vi "Initialize Sessions.vi"(0 "Session Handle in":T1, 5 "Baud Rate":u32=250000, 7 "Termination":u32(ring)=1 items=["Off", "On"], 11 "error in (no error)":errorcluster) -> (4 "Session Handle Out":T1, 15 "error out":errorcluster)   [LabVIEW 2015, in "PAS.lvclass"]
uses:
  PAS.lvclass
  Typedefs/Session Handle.ctl
  PAS.lvclass/PAS.ctl
  <vilib>/xnet/xnet.llb/XNET Create Session (Frame Output Stream).vi
  <vilib>/xnet/xnet.llb/XNET Create Session (Frame Input Stream).vi
  <resource>/objmgr/xnet.rc
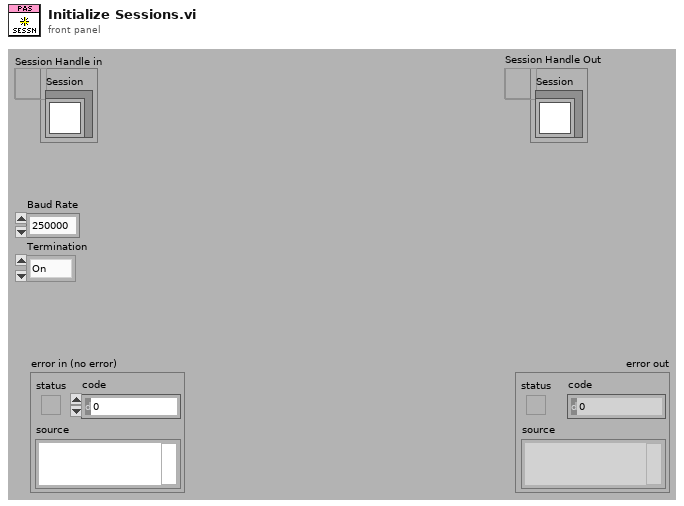
[diagram p1: front panel]
types:
  T1 = typedef "PAS.lvclass/Session Handle.ctl" = refnum<data-value>
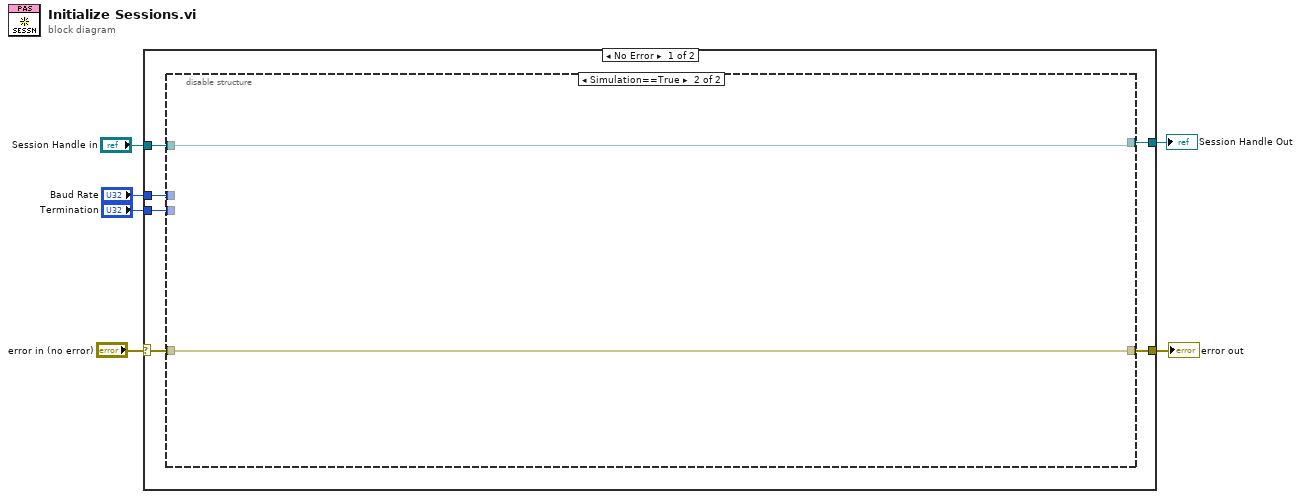
[diagram p0: block diagram]
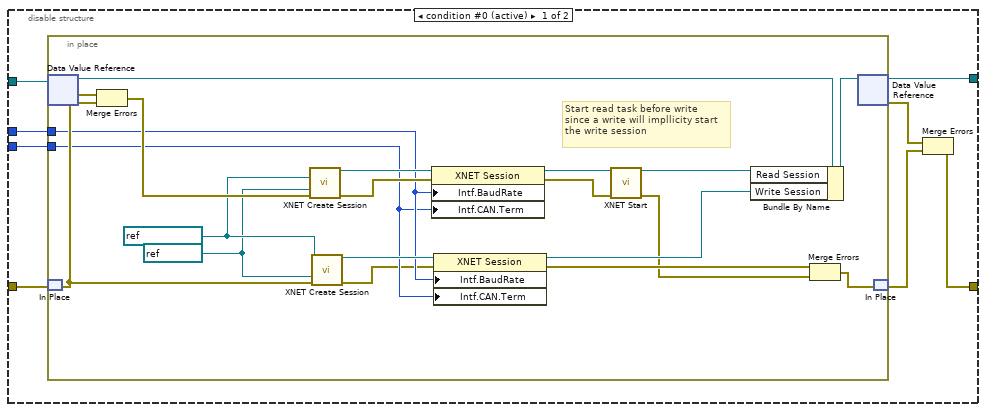
[diagram p2: hidden frame]
diagram:
  n1 = case shown="No Error" "error in (no error)" {
    selector: "error in (no error)" -> [w11 w44]
    tunnel: [w12 w44] -> w6
    tunnel: "Baud Rate" -> [w10 _]
    tunnel: "Termination" -> [w9 _]
    tunnel: "Session Handle in" -> [w8 w43]
    tunnel: [w7 w43] -> w1
    frame No Error {
      n2 = disable-structure shown="Simulation==True" {
        disable-tunnel: [w18 w41] -> w12
        disable-tunnel: w11 -> [w17 w41]
        disable-tunnel: w10 -> [w16 _]
        disable-tunnel: w9 -> [w15 _]
        disable-tunnel: w8 -> [w14 w42]
        disable-tunnel: [w13 w42] -> w7
        frame condition #0 (active) {
          n3 = in-place {
            in-place-border: w16 -> [w32]
            in-place-border: w15 -> [w31]
            w37 = refnum<k21> "CAN1" ("Select Interface")
            w38 = refnum<k21> ":memory:" ("CAN Cluster")
            # "Start read task before write\nsince a write will impllicity start\nthe write session"
            n4 = in-place-dvr #1(w14) -> (w22:refnum<class "PAS.lvclass">, w40:errorcluster)
            n5 = in-place-match #2(w17) -> (w36:errorcluster)
            n6 = Merge Errors(w36, w40) -> (w39:errorcluster)
            n7 = call-poly <vilib>:"XNET Create Session.vi"("cluster (:memory:)"=w38, "interface"=w37, "error in (no error)"=w39) -> ("session out"=w35:refnum<k21>, "error out"=w34:errorcluster)  [unwired: 11 out]
            n8 = call-poly <vilib>:"XNET Create Session.vi"("cluster (:memory:)"=w38, "interface"=w37, "error in (no error)"=w36) -> ("session out"=w33:refnum<k21>, "error out"=w30:errorcluster)  [unwired: 11 out]
            n9 = property class="XNET Session"(reference=w35, error in=w34, "Intf.BaudRate"=w32, "Intf.CAN.Term"=w31) -> (reference out=w26:refnum<k21>, error out=w25:errorcluster)
            n10 = property class="XNET Session"(reference=w33, error in=w30, "Intf.BaudRate"=w32, "Intf.CAN.Term"=w31) -> (reference out=w29:refnum<k21>, error out=w28:errorcluster)
            n11 = call <vilib>:"XNET Start.vi"("session in"=w26, "error in (no error)"=w25) -> ("session out"=w24:refnum<k21>, "error out"=w23:errorcluster)  [unwired: 12 in]
            n12 = Bundle By Name(cluster=w22, "Read Session"=w24, "Write Session"=w29) -> (w21:refnum<class "PAS.lvclass">)
            n13 = Merge Errors(w28, w23) -> (w27:errorcluster)
            n14 = in-place-dvr #1(w21) -> (w13:T1, w19:errorcluster)
            n15 = in-place-match #2(w27) -> (w20:errorcluster)
          }
          n16 = Merge Errors(w19, w20) -> (w18:errorcluster)
        }
        frame condition #1 {
        }
      }
    }
    frame Error {
    }
  }
  "error out" <- w6
  "Session Handle Out" <- w1
